vi "CONST ErrorDefinitions.vi"() -> (1 "Error Descriptions":string[](array[string]), 2 "Error Titles":string[](array[string]), 3 "Error Codes":i32[](array[numeric]))   [LabVIEW 2013, in "LapDog.Collections.v1.Common.lvlib"]
uses:
  LapDog.Collections.v1.Common.lvlib
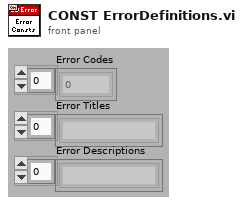
[diagram p1: front panel]
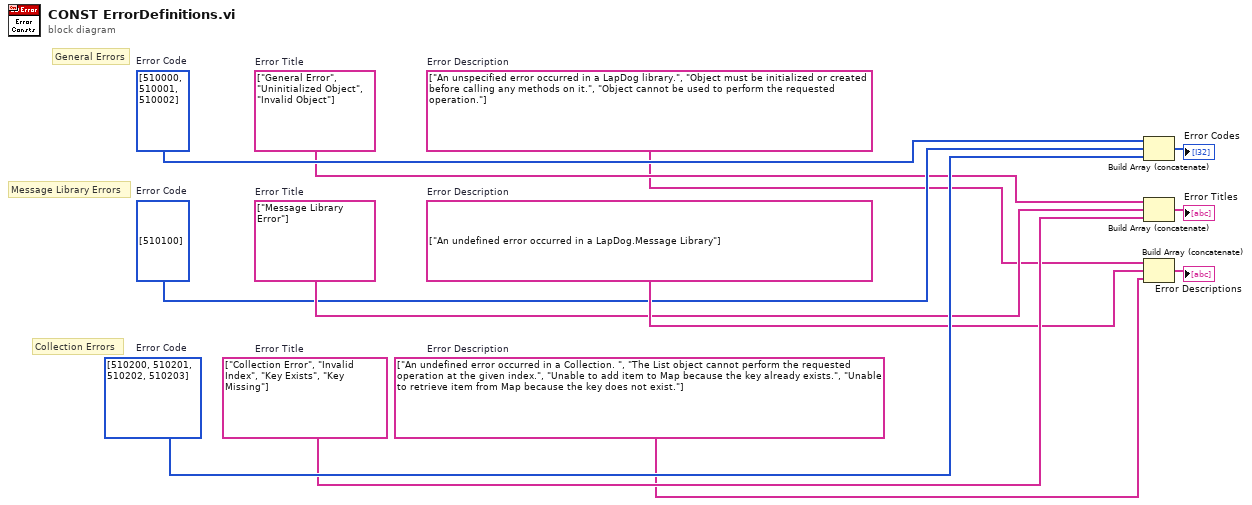
[diagram p0: block diagram]
diagram:
  w9 = string[] ["An undefined error occurred in a LapDog.Message Library"]  # Error Description
  w7 = i32[] [510100]  # Error Code
  w8 = string[] ["Message Library Error"]  # Error Title
  w10 = string[] ["An undefined error occurred in a Collection. ", "The List object cannot perform the requested operation at the given index.", "Unable to add item to Map because the key already exists.", "Unable to retrieve item from Map because the key does not exist."]  # Error Description
  w12 = i32[] [510200, 510201, 510202, 510203]  # Error Code
  w11 = string[] ["Collection Error", "Invalid Index", "Key Exists", "Key Missing"]  # Error Title
  w4 = string[] ["An unspecified error occurred in a LapDog library.", "Object must be initialized or created before calling any methods on it.", "Object cannot be used to perform the requested operation."]  # Error Description
  w6 = i32[] [510000, 510001, 510002]  # Error Code
  w5 = string[] ["General Error", "Uninitialized Object", "Invalid Object"]  # Error Title
  # "Message Library Errors"
  # "Collection Errors"
  # "General Errors"
  n1 = Build Array (concatenate)(w6, w7, w12) -> (→"Error Codes":i32[])
  n2 = Build Array (concatenate)(w5, w8, w11) -> (→"Error Titles":string[])
  n3 = Build Array (concatenate)(w4, w9, w10) -> (→"Error Descriptions":string[])
